vi "LVDeleteFile_Item_OnPopupMenu.vi"(11 "Object":T1) -> ()   [LabVIEW 2018]
uses:
  <resource>/Framework/Providers/API/mxLvMenuItem.ctl
  <resource>/Framework/Providers/API/ItemRef.ctl
panel:
  out "error out":errorcluster
  in  "error in":errorcluster
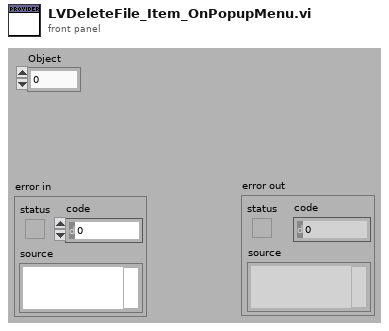
[diagram p1: front panel]
types:
  T1 = typedef "ItemRef.ctl" = u64
  T2 = typedef "mxLvMenuItem.ctl" = cluster{"Menu Name":string, "Description":string, "Icon File Name":path, "Menu Tag":string, "Enabled":bool, "Checked":bool, "Separator":bool, "Batchable":bool, "Weight":i32, "Batch Mode (Ignored if Not Batchable)":enum32{"Show If All Items Support Command", "Show If Any Items Support Command"}, "Menu Location":enum32{"<None>", "Project", "Project / Build Specifications", "Tools", "Tools / Source Control", "Tools / Real-Time Module", "Help"}, "Exclude From Getting Started Window Menu":bool}
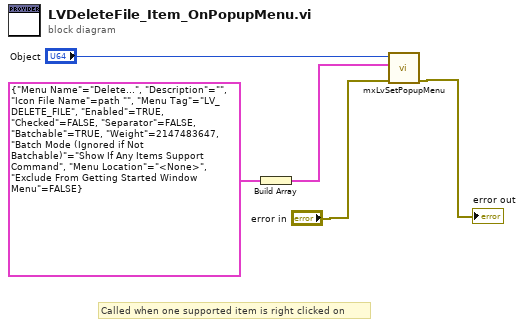
[diagram p0: block diagram]
diagram:
  # "Called when one supported item is right clicked on"
  n1 = Build Array(T2 {"Menu Name"="Delete...", "Description"="", "Icon File Name"=path "", "Menu Tag"="LV_DELETE_FILE", "Enabled"=TRUE, "Checked"=FALSE, "Separator"=FALSE, "Batchable"=TRUE, "Weight"=2147483647, "Batch Mode (Ignored if Not Batchable)"=enum."Show If Any Items Support Command", "Menu Location"=enum."<None>", "Exclude From Getting Started Window Menu"=FALSE} ("Menu Item")) -> (w4:T2[])
  n2 = call <resource>:"mxLvSetPopupMenu.vi"("error in"="error in", "Popup Menu Items"=w4, "Item"="Object") -> ("error out"=→"error out":errorcluster)  [unwired: 7 in, 1 out]
